vi "Untitled 2.vi"() -> ()   [LabVIEW 2017]
uses:
  5119f692-16e2-4fa7-a502-6bcaf288f741.vi
  9438c21e-99d4-4d36-a3b1-840b035dd6a9.vi
  5119f692-16e2-4fa7-a502-6bcaf288f741.vi/b09b9099-6be0-413b-8afc-4908471460c3.vi
  9438c21e-99d4-4d36-a3b1-840b035dd6a9.vi/b09b9099-6be0-413b-8afc-4908471460c3.vi
  INI-Static-Variable-Support/_Support/global-csm-ini-db-change-flag.vi
  <vilib>/Utility/Data Type/Get Type Information.vi
  <userlib>/_NEVSTOP/Communicable State Machine(CSM)/addons/API-String-Arugments-Support/_Support/Data To SingleElementsArray_csm.vi
  INI-Static-Variable-Support/_Support/Parse Used Session and Name.vi
  <userlib>/_NEVSTOP/Communicable State Machine(CSM)/addons/API-String-Arugments-Support/_Support/Data To API String Arguments.vi
  INI-Static-Variable-Support/_Support/INI-FGV.vi
  <userlib>/_NEVSTOP/Communicable State Machine(CSM)/addons/API-String-Arugments-Support/_Support/Convert API String Arguments to Data(variant).vi
  <userlib>/_NEVSTOP/Communicable State Machine(CSM)/addons/API-String-Arugments-Support/_Support/SingleElementsArray To Data_csm.vi
  INI-Static-Variable-Support/INI-Static-Variable-Support.lvlib
panel:
  out "String out":string
  out "config out 2":cluster{"Enable":bool, "Path":path}
  out "error out":errorcluster
  out "config out":bool
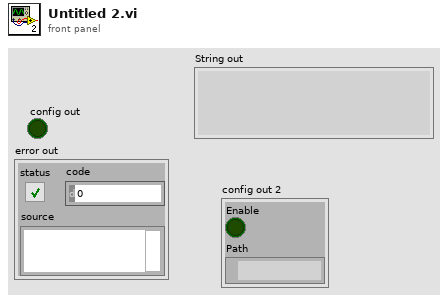
[diagram p1: front panel]
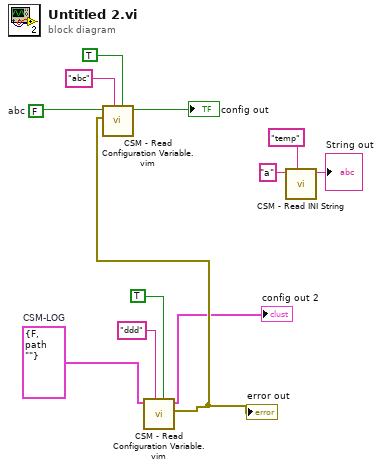
[diagram p0: block diagram]
diagram:
  w8 = cluster{"Enable":bool, "Path":path} {"Enable"=FALSE, "Path"=path ""}  # CSM-LOG
  w9 = FALSE  # abc
  n1 = call "CSM - Read Configuration Variable.vim"("Write If not found?(F)"=TRUE, "Section Name(\"\" as Default)"="ddd" ("Section Name(\"\" as Default)"), "config prototype(Cluster Prefered)"=w8) -> ("error out"=w5:errorcluster, "config out"=→"config out 2":cluster{"Enable":bool, "Path":path})  [unwired: 5 in]
  "error out" <- w5
  n2 = call "CSM - Read Configuration Variable.vim"("Write If not found?(F)"=TRUE, "Section Name(\"\" as Default)"="abc" ("Section Name(\"\" as Default)"), "error in (no error)"=w5, "config prototype(Cluster Prefered)"=w9) -> ("config out"=→"config out":bool)  [unwired: 4 in, 1 out]
  n3 = call "CSM - Read INI String.vi"("Section Name(\"\" as Default)"="temp" ("Section Name(\"\" as Default)"), "String in"="a") -> ("String out"=→"String out":string)  [unwired: 5 in, 2 out]
